vi "Load Config.vi"(8 "error in (no error)":errorcluster, 11 "Data Logger Module in":refnum<class "Data Logger Module.lvclass">) -> (0 "error out":errorcluster, 3 "Data Logger Module out":refnum<class "Data Logger Module.lvclass">)   [LabVIEW 2020, in "VolatusData.lvlib" / "Data Logger Module.lvclass"]
uses:
  Data Logger Module.lvclass
  Data Logger Module.lvclass/Data Logger Module.ctl
  Volatus/Module/Module.lvclass
  VolatusConfig/VolatusConfigElement/VolatusConfigElement.lvclass
  lv-cdm/CDM-Config/Config Element/Config Element.lvclass
  C:/dev/lv20CE/relink/lv-volatus/Volatus/Module/Module.lvclass
  C:/dev/lv20CE/relink/lv-volatus/VolatusData/Data Logger Module/Data Logger Module.lvclass
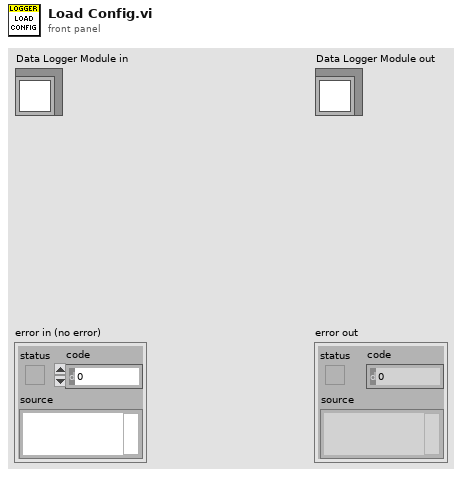
[diagram p1: front panel]
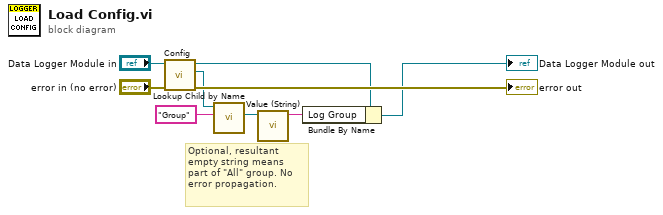
[diagram p0: block diagram]
diagram:
  # "Optional, resultant empty string means part of \"All\" group. No error propagation."
  n1 = call "Config.vi"("Module in"="Data Logger Module in") -> ("Config"=w5:refnum<class "VolatusConfigElement.lvclass">, "Module out"=w6:refnum<class "Data Logger Module.lvclass">)  [unwired: 9 in]
  n2 = call "Lookup Child by Name.vi"("Child Name"="Group", "VolatusConfigElement in"=w5) -> ("Child"=w3:refnum<class "Config Element.lvclass">)  [unwired: 6 in, 3 out]
  n3 = call "Value (String).vi"("Config Element in"=w3) -> ("String Value"=w1:string)  [unwired: 9 in, 1 out]
  n4 = Bundle By Name(cluster=w6, "Log Group"=w1) -> (→"Data Logger Module out":refnum<class "Data Logger Module.lvclass">)
  "error out" <- "error in (no error)"
